vi "Actor Core.vi"(8 "error in":errorcluster, 11 "Main View in":refnum<class "Main View.lvclass">) -> (0 "error out":errorcluster, 3 "Actor out":refnum<class "Actor.lvclass">)   [LabVIEW 2020, in "Main View.lvlib" / "Main View.lvclass"]
doc: "(<B>Filename</B>: Actor Framework.lvlib:Actor.lvclass:Actor Core.vi)\n\nReceives messages to the actor, reacts to them, and initiates any error handling that may shut the actor down.\n\nDescendant classes may override this VI to append parallel tasks for the actor to complete while it handles messages. Overrides use the Call Parent Method node."
uses:
  Main View.lvclass
  C:/Program Files/National Instruments/LabVIEW 2020/vi.lib/ActorFramework/Actor/Actor.lvclass
  <vilib>/ActorFramework/Actor/Actor.lvclass
  <vilib>/ActorFramework/Actor/Actor.lvclass/Actor.ctl
  Main View.lvclass/Main View.ctl
  <vilib>/ActorFramework/Message Enqueuer/Message Enqueuer.lvclass/Message Enqueuer.ctl
  <vilib>/ActorFrameworkMVC/View Controller/View Controller Messages/Set Subpanel Msg/Set Subpanel Msg.lvclass/Set Subpanel Msg.ctl
  Controllers/UI Controller/UI Controller Messages/Resize Subpanel Msg/Resize Subpanel Msg.lvclass/Resize Subpanel Msg.ctl
  Controllers/UI Controller/UI Controller Messages/Update Main View Msg/Update Main View Msg.lvclass/Update Main View Msg.ctl
  Controllers/UI Controller/UI Controller Messages/Register Datum When Mouse Down Msg/Register Datum When Mouse Down Msg.lvclass/Register Datum When Mouse Down Msg.ctl
  <vilib>/ActorFramework/Message Enqueuer/Init from Existing Queue.vi
  <vilib>/ActorFramework/Message Enqueuer/Enqueue.vi
  <vilib>/ActorFrameworkMVC/View Controller/View Controller Messages/Set Subpanel Msg/Set Subpanel Msg.lvclass
  C:/Program Files/National Instruments/LabVIEW 2020/vi.lib/ActorFramework/Message/Message.lvclass
  Controllers/UI Controller/UI Controller Messages/Resize Subpanel Msg/Resize Subpanel Msg.lvclass
  Controllers/UI Controller/UI Controller Messages/Update Occupied Area Msg/Update Occupied Area Msg.lvclass
  Controllers/UI Controller/UI Controller Messages/Update Main View Msg/Update Main View Msg.lvclass
  Controllers/UI Controller/UI Controller Messages/Register Datum When Mouse Down Msg/Register Datum When Mouse Down Msg.lvclass
  <vilib>/ActorFramework/Stop Msg/Stop Msg.lvclass
  <vilib>/ActorFramework/Message Priority Queue/Priority Enqueue.vi
  <vilib>/ActorFramework/Message Enqueuer/Message Enqueuer.lvclass
  <vilib>/ActorFrameworkMVC/Abstract View/Abstract View/Abstract View.lvclass
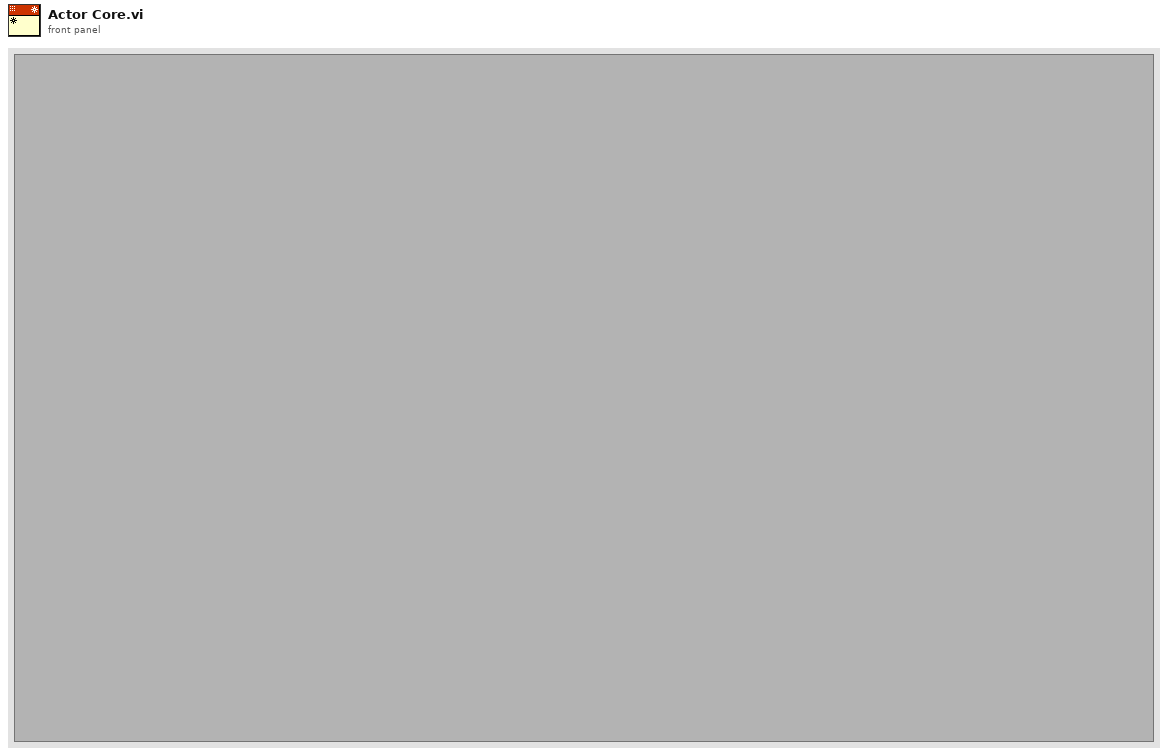
[diagram p1: front panel]
types:
  T1 = typedef "LVRectTypeDef.ctl" = cluster{"Left":i16, "Top":i16, "Right":i16, "Bottom":i16}
  T2 = typedef "LVPoint32TypeDef.ctl" = cluster{"Horizontal":i32, "Vertical":i32}
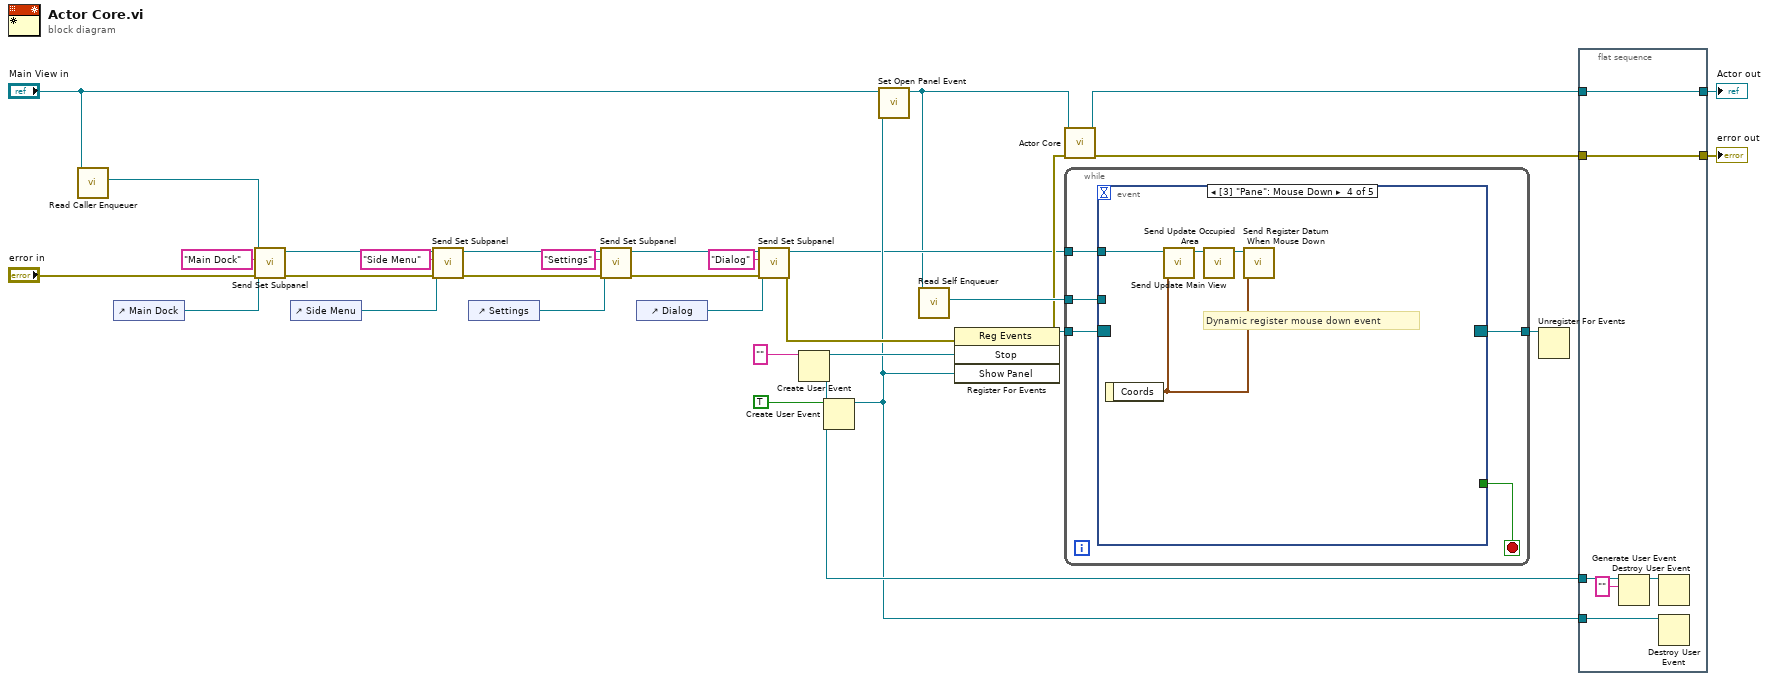
[diagram p0: block diagram]
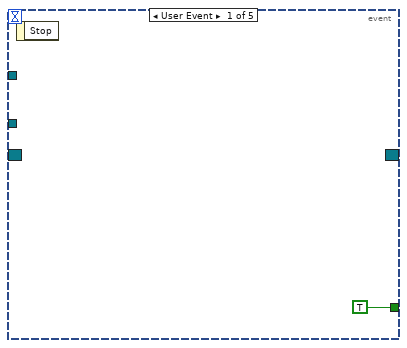
[diagram p2: hidden frame]
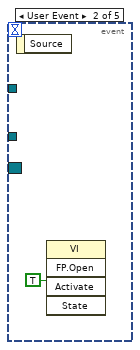
[diagram p3: hidden frame]
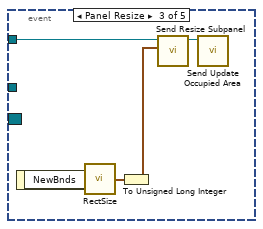
[diagram p4: hidden frame]
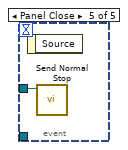
[diagram p5: hidden frame]
diagram:
  n1 = call <vilib>:"Read Caller Enqueuer.vi"("Actor"="Main View in") -> ("Caller Enqueuer"=w25:refnum<class "Message Enqueuer.lvclass">)  [unwired: 10 in]
  n2 = control-ref of="Main Dock"() -> (w20:refnum<vi>)
  n3 = call <vilib>:"Send Set Subpanel.vi"("error in (no error)"="error in", "SubPanel Reference"=w20, "Subpanel Name"="Main Dock", "Message Enqueuer"=w25) -> ("error out"=w24:errorcluster, "Message Enqueuer out"=w32:refnum<class "Message Enqueuer.lvclass">)  [unwired: 6 in]
  n4 = control-ref of="Side Menu"() -> (w4:refnum<vi>)
  n5 = call <vilib>:"Send Set Subpanel.vi"("error in (no error)"=w24, "SubPanel Reference"=w4, "Subpanel Name"="Side Menu", "Message Enqueuer"=w32) -> ("error out"=w22:errorcluster, "Message Enqueuer out"=w26:refnum<class "Message Enqueuer.lvclass">)  [unwired: 6 in]
  n6 = control-ref of="Settings"() -> (w3:refnum<vi>)
  n7 = call <vilib>:"Send Set Subpanel.vi"("error in (no error)"=w22, "SubPanel Reference"=w3, "Subpanel Name"="Settings", "Message Enqueuer"=w26) -> ("error out"=w21:errorcluster, "Message Enqueuer out"=w27:refnum<class "Message Enqueuer.lvclass">)  [unwired: 6 in]
  n8 = control-ref of="Dialog"() -> (w2:refnum<vi>)
  n9 = call <vilib>:"Send Set Subpanel.vi"("error in (no error)"=w21, "SubPanel Reference"=w2, "Subpanel Name"="Dialog", "Message Enqueuer"=w27) -> ("error out"=w11:errorcluster, "Message Enqueuer out"=w5:refnum<class "Message Enqueuer.lvclass">)  [unwired: 6 in]
  n10 = Create User Event(user event datatype="" ("Stop")) -> (user event=w14:refnum<user-event>)  [unwired: 1 in, 1 out]
  n11 = Create User Event(user event datatype=TRUE ("Show Panel")) -> (user event=w10:refnum<user-event>)  [unwired: 1 in, 1 out]
  n12 = call "Set Open Panel Event.vi"("Show Panel Event"=w10, "Main View in"="Main View in") -> ("Main View out"=w1:refnum<class "Main View.lvclass">)  [unwired: 9 in]
  n13 = call <vilib>:"Read Self Enqueuer.vi"("Actor"=w1) -> ("Self Enqueuer"=w15:refnum<class "Message Enqueuer.lvclass">)  [unwired: 10 in]
  n14 = register-events(error in=w11, w14, w10) -> (reference out=w16:refnum<event-registration>, error out=w9:errorcluster)  [unwired: 1 in]
  n15 = call-parent "Actor Core.vi"("error in"=w9, "Abstract View in"=w1) -> ("error out"=w8:errorcluster, "Actor out"=w13:refnum<class "Actor.lvclass">)  [unwired: 8 in]
  n16 = while {
    tunnel: w16 -> [w37]
    tunnel: [w36] -> w17
    tunnel: w15 -> [w34]
    tunnel: w5 -> [w33]
    stop <- w35 stop-if-true
    n17 = event shown="[3] \"Pane\": Mouse Down" {
      selector: w37 -> [_ _ _ _ _]
      dyn-events: [_ _ _ _ _] -> w36
      timeout: _ -> [_ _ _ _ _]
      tunnel: [TRUE _ _ _ _] -> w35
      tunnel: w34 -> [_ _ _ _ _]
      tunnel: w33 -> [_ _ w42 w48 w49]
      event User Event {
        n18 = event-data() -> ()  [unwired: 1 in, 1 out]
      }
      event User Event {
        n19 = event-data() -> ()  [unwired: 1 in, 1 out]
        n20 = invoke class="VI" method="FP.Open"("Activate"=TRUE ("Activate?")) -> ()  [unwired: 4 in, 5 out]
      }
      event Panel Resize {
        n21 = event-data() -> ("NewBnds"=w43:T1)  [unwired: 1 in]
        n22 = call <vilib>:"RectSize.vi"("rect"=w43) -> ("point"=w44:cluster{"x":i16, "y":i16})
        n23 = To Unsigned Long Integer(number=w44) -> (unsigned 32bit integer=w40:cluster{"x":u32, "y":u32})
        n24 = call "Send Resize Subpanel.vi"("Subpanel Size"=w40, "Message Enqueuer"=w42) -> ("Message Enqueuer out"=w41:refnum<class "Message Enqueuer.lvclass">)  [unwired: 8 in, 1 out]
        n25 = call "Send Update Occupied Area.vi"("Message Enqueuer"=w41) -> ()  [unwired: 9 in, 2 out]
      }
      event Mouse Down {
        # "Dynamic register mouse down event"
        n26 = event-data() -> ("Coords"=w47:T2)  [unwired: 1 in]
        n27 = call "Send Update Main View.vi"("Position"=w47, "Message Enqueuer"=w48) -> ("Message Enqueuer out"=w46:refnum<class "Message Enqueuer.lvclass">)  [unwired: 8 in, 1 out]
        n28 = call "Send Update Occupied Area.vi"("Message Enqueuer"=w46) -> ("Message Enqueuer out"=w45:refnum<class "Message Enqueuer.lvclass">)  [unwired: 9 in, 1 out]
        n29 = call "Send Register Datum When Mouse Down.vi"("Position"=w47, "Message Enqueuer"=w45) -> ()  [unwired: 8 in, 2 out]
      }
      event Panel Close {
        n30 = event-data() -> ()  [unwired: 1 in, 1 out]
        n31 = call <vilib>:"Send Normal Stop.vi"("Message Enqueuer"=w49) -> ()  [unwired: 10 in, 1 out]
      }
    }
  }
  n32 = Unregister For Events(event registration refnum=w17) -> ()  [unwired: 1 in, 1 out]
  n33 = flat-sequence {
    tunnel: w14 -> [w54]
    tunnel: w10 -> [w52]
    tunnel: w13 -> [w51]
    tunnel: [w51] -> w6
    tunnel: [w50] -> w7
    tunnel: w8 -> [w50]
    frame #0 {
      n34 = Generate User Event(user event=w54, event data cluster="" ("event data")) -> (user event out=w55:refnum<user-event>)  [unwired: 2 in, 1 out]
      n35 = Destroy User Event(user event=w55) -> ()  [unwired: 1 in, 1 out]
      n36 = Destroy User Event(user event=w52) -> ()  [unwired: 1 in, 1 out]
    }
  }
  "error out" <- w7
  "Actor out" <- w6
